vi "ResultSavePrompt.vi"(0 "Path":path) -> (1 "selected path":path, 2 "cancel?":bool)   [LabVIEW 2024]
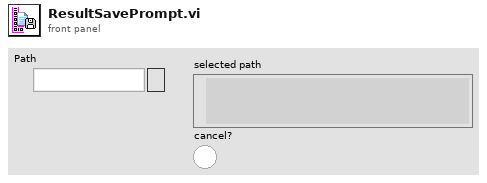
[diagram p1: front panel]
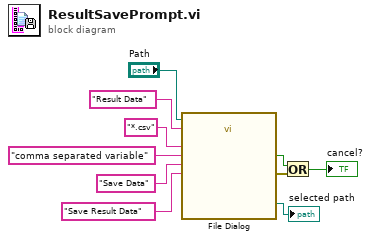
[diagram p0: block diagram]
diagram:
  n1 = call "File Dialog"("start path"="Path", "prompt"="Save Result Data", "button label"="Save Data", "default name"="Result Data", "pattern (all files)"="*.csv", "pattern label"="comma separated variable") -> ("selected path"=→"selected path":path, "cancelled"=w9:bool, "error out"=w10:errorcluster)  [unwired: 6 in, 1 out]
  n2 = Or(x=w9, y=w10) -> (x .or. y?=→"cancel?":bool)
